vi "Snap to Center.vi"(9 "Fixed Rect":T1, 11 "Rect":T1) -> (1 "TopLeft point":cluster{"x":i32, "y":i32}, 3 "Snapped to center":T1)   [LabVIEW 2012]
doc: "This VI calculates the position of a snapped-to-left rectangle from the positions of a large rectangle and a smaller one that will be positioned inside."
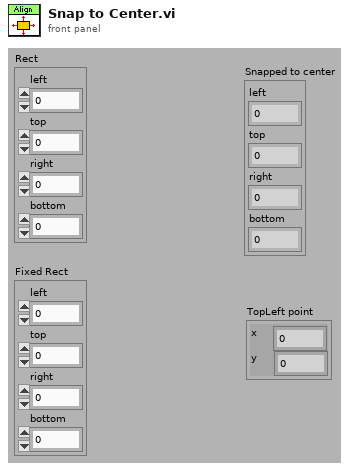
[diagram p1: front panel]
types:
  T1 = cluster{"left":i16, "top":i16, "right":i16, "bottom":i16}
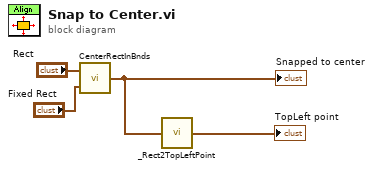
[diagram p0: block diagram]
diagram:
  n1 = call <vilib>:"CenterRectInBnds.vi"("bounds"="Fixed Rect", "rect"="Rect") -> ("centered rect"=w2:T1)
  "Snapped to center" <- w2
  n2 = call "_Rect2TopLeftPoint.vi"("bounds"=w2) -> ("TopLeft point"=→"TopLeft point":cluster{"x":i32, "y":i32})  [unwired: 4 out]
